vi "Initilaize Views.vi"(8 "error in (no error)":errorcluster, 11 "Controller in":refnum<class "Controller.lvclass">) -> (0 "error out":errorcluster, 3 "Controller out":refnum<class "Controller.lvclass">)   [LabVIEW 2023, in "MVC Actors.lvlib" / "Controller.lvclass"]
doc: "This abstract dynamic dispatch VI has to be overridden by the concrete Controller Actor subclasses in order to initialize the View Actors that are going to register for events. Within the concrete implementation of this abstract method the user will call the <b>Add View.vi</b> method for each of the <b>Views</b> to be initialized. This method is automatically executed upon Controller launch, other events can be dynamically defined during the Controller execution by calling the <b>Add View.vi</b> method."
uses:
  Controller.lvclass
  Controller.lvclass/Controller.ctl
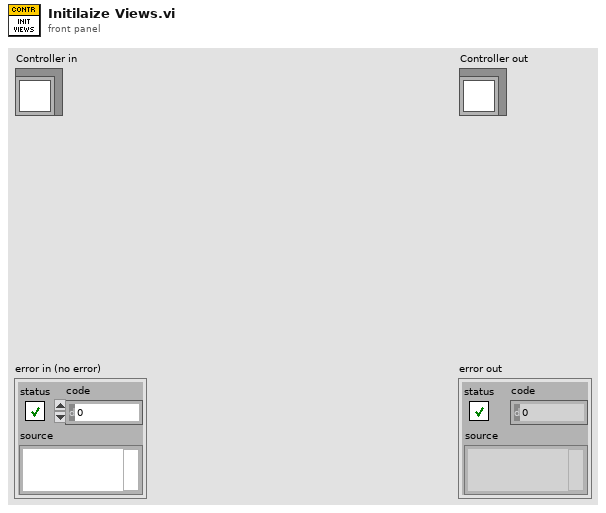
[diagram p1: front panel]
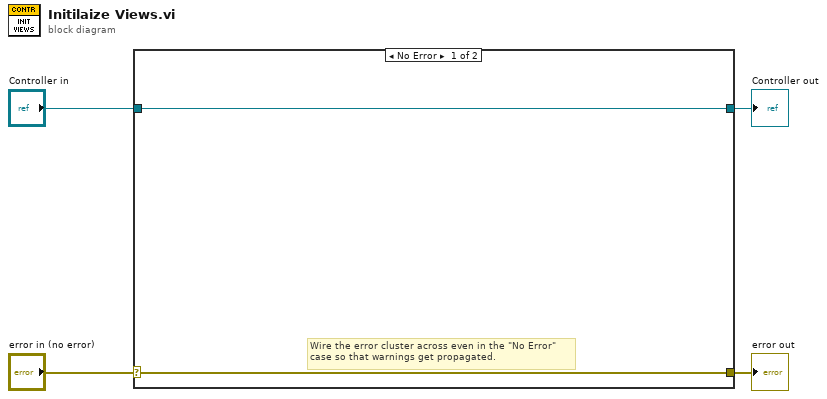
[diagram p0: block diagram]
diagram:
  n1 = case shown="No Error" "error in (no error)" {
    selector: "error in (no error)" -> [w5 w8]
    tunnel: [w5 w8] -> w3
    tunnel: [w6 w7] -> w1
    tunnel: "Controller in" -> [w6 w7]
    frame No Error {
      # "Wire the error cluster across even in the \"No Error\"\ncase so that warnings get propagated."
    }
    frame Error {
    }
  }
  "error out" <- w3
  "Controller out" <- w1
